vi "Post-Install Custom Action.vi"(10 "Variant":variant) -> (0 "error out":errorcluster)   [LabVIEW 2013]
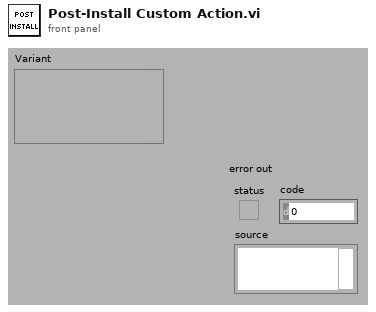
[diagram p1: front panel]
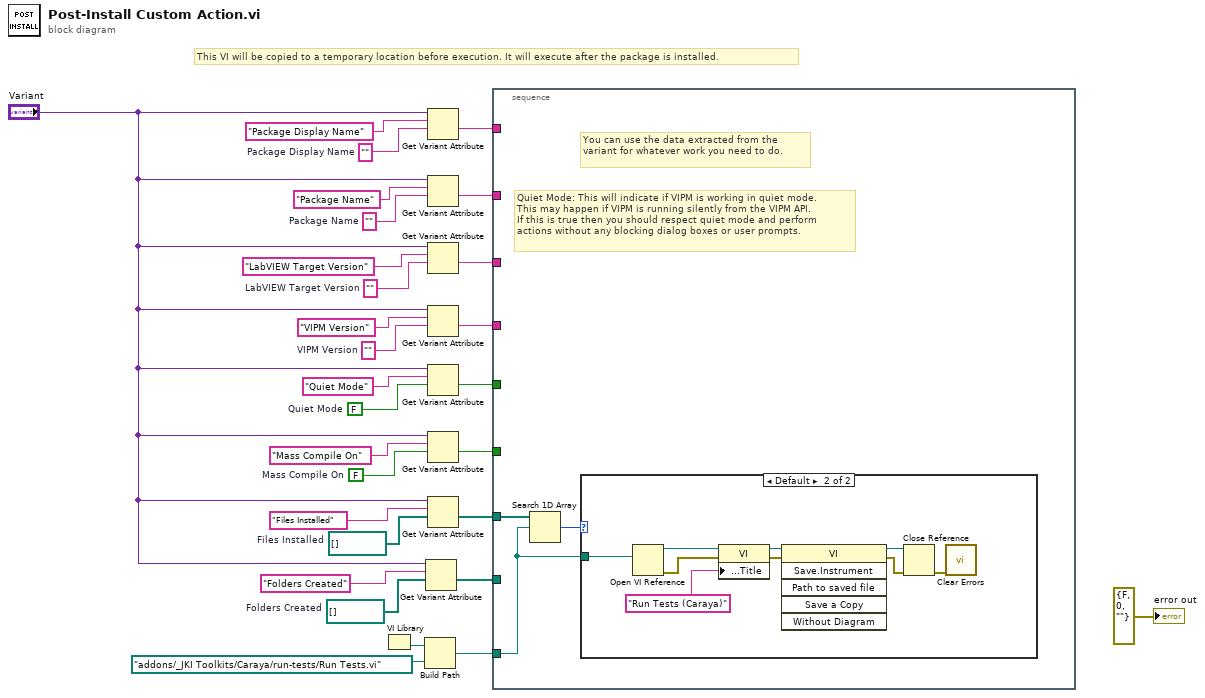
[diagram p0: block diagram]
diagram:
  w4 = path[] []  # Folders Created
  w5 = path[] []  # Files Installed
  w11 = FALSE  # Mass Compile On
  w12 = ""  # Package Display Name
  w19 = FALSE  # Quiet Mode
  w22 = ""  # VIPM Version
  w24 = ""  # LabVIEW Target Version
  w26 = ""  # Package Name
  # "This VI will be copied to a temporary location before execution. It will execute after the package is installed."
  n1 = VI Library() -> (path=w3:path)
  n2 = Build Path(base path=w3, name or relative path=path "addons/_JKI Toolkits/Caraya/run-tests/Run Tests.vi") -> (appended path=w1:path)
  n3 = Get Variant Attribute(Variant="Variant", name="Folders Created", default value (empty Variant)=w4) -> (value=w9:path[])  [unwired: 1 in, 3 out]
  n4 = Get Variant Attribute(Variant="Variant", name="Package Display Name", default value (empty Variant)=w12) -> (value=w18:string)  [unwired: 1 in, 3 out]
  n5 = Get Variant Attribute(Variant="Variant", name="Package Name", default value (empty Variant)=w26) -> (value=w17:string)  [unwired: 1 in, 3 out]
  n6 = Get Variant Attribute(Variant="Variant", name="LabVIEW Target Version", default value (empty Variant)=w24) -> (value=w16:string)  [unwired: 1 in, 3 out]
  n7 = Get Variant Attribute(Variant="Variant", name="VIPM Version", default value (empty Variant)=w22) -> (value=w15:string)  [unwired: 1 in, 3 out]
  n8 = Get Variant Attribute(Variant="Variant", name="Quiet Mode", default value (empty Variant)=w19) -> (value=w14:bool)  [unwired: 1 in, 3 out]
  n9 = Get Variant Attribute(Variant="Variant", name="Mass Compile On", default value (empty Variant)=w11) -> (value=w13:bool)  [unwired: 1 in, 3 out]
  n10 = Get Variant Attribute(Variant="Variant", name="Files Installed", default value (empty Variant)=w5) -> (value=w8:path[])  [unwired: 1 in, 3 out]
  n11 = stacked-sequence {
    tunnel: w18 -> [_]
    tunnel: w17 -> [_]
    tunnel: w16 -> [_]
    tunnel: w15 -> [_]
    tunnel: w14 -> [_]
    tunnel: w13 -> [_]
    tunnel: w8 -> [w32]
    tunnel: w9 -> [_]
    tunnel: w1 -> [w30]
    frame #0 {
      # "Quiet Mode: This will indicate if VIPM is working in quiet mode.\nThis may happen if VIPM is running silently from the VIPM API.\nIf this is true then you should respect quiet mode and perform\nactions without any blocking dialog boxes or user prompts."
      # "You can use the data extracted from the variant for whatever work you need to do."
      n12 = Search 1D Array(1D array=w32, element=w30) -> (index of element=w31:i32)  [unwired: 1 in]
      n13 = case shown="Default" w31 {
        tunnel: w30 -> [_ w41]
        frame -1 {
        }
        frame Default {
          n14 = Open VI Reference(vi path=w41) -> (vi reference=w40:refnum<vi>, error out=w38:errorcluster)  [unwired: 5 in]
          n15 = property class="VI"(reference=w40, error in=w38, "Front Panel.Title"="Run Tests (Caraya)") -> (reference out=w37:refnum<vi>, error out=w36:errorcluster)
          n16 = invoke class="VI" method="Save.Instrument"(reference=w37, error in=w36) -> (reference out=w34:refnum<vi>, error out=w35:errorcluster)  [unwired: 4 in, 4 out]
          n17 = Close Reference(reference=w34, error in (no error)=w35) -> (error out=w33:errorcluster)
          n18 = call <vilib>:"Clear Errors.vi"("error in (no error)"=w33) -> ()  [unwired: 6 in, 1 out]
        }
      }
    }
  }
  "error out" <- errorcluster {"status"=FALSE, "code"=0, "source"=""} ("error out")
